vi "bone it.vi"() -> ()   [LabVIEW 2015]
panel:
  in  "milliseconds to wait 2":u32
  in  "milliseconds to wait":u32
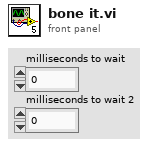
[diagram p1: front panel]
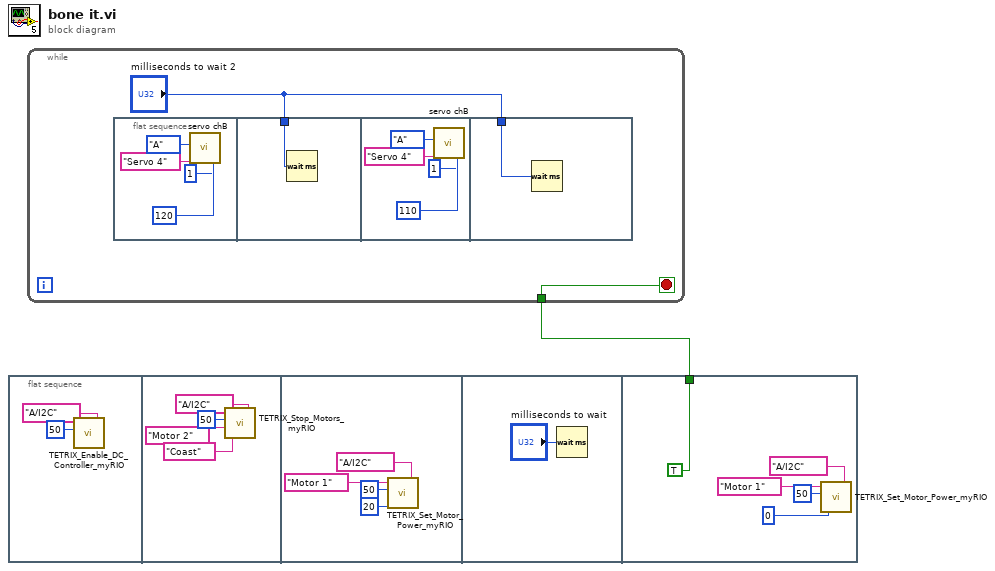
[diagram p0: block diagram]
diagram:
  n1 = flat-sequence {
    tunnel: [TRUE] -> w1
    frame #0 {
      n2 = call <vilib>:"TETRIX_Enable_DC_Controller_myRIO.vi"("myRIO MXP Port A/B"=tag "A/I2C", "Controller ID#  (I2C Address)"=u8 50) -> ()  [unwired: 5 in, 1 out]
    }
    frame #1 {
      n3 = call <vilib>:"TETRIX_Stop_Motors_myRIO.vi"("myRIO MXP Port A/B"=tag "A/I2C", "Stop Mode"="Coast", "Select Channel"="Motor 2", "Controller ID#  (I2C Address)"=u8 50) -> ()  [unwired: 3 in, 1 out]
    }
    frame #2 {
      n4 = call <vilib>:"TETRIX_Set_Motor_Power_myRIO.vi"("myRIO MXP Port A/B"=tag "A/I2C", "Power (-100 to 100)  0 = Coast Stop  125 = Brake Stop"=i8 20, "Select Channel"="Motor 1", "Controller ID#  (I2C Address)"=u8 50) -> ()  [unwired: 3 in, 1 out]
    }
    frame #3 {
      n5 = Wait (ms)(milliseconds to wait="milliseconds to wait") -> ()  [unwired: 1 out]
    }
    frame #4 {
      n6 = call <vilib>:"TETRIX_Set_Motor_Power_myRIO.vi"("myRIO MXP Port A/B"=tag "A/I2C", "Power (-100 to 100)  0 = Coast Stop  125 = Brake Stop"=i8 0, "Select Channel"="Motor 1", "Controller ID#  (I2C Address)"=u8 50) -> ()  [unwired: 3 in, 1 out]
    }
  }
  n7 = while {
    tunnel: w1 -> [w19]
    stop <- w19 stop-if-true
    n8 = flat-sequence {
      tunnel: "milliseconds to wait 2" -> [w24]
      tunnel: "milliseconds to wait 2" -> [w29]
      frame #0 {
        n9 = call "servo chB.vi"("Servo Position (0 - 255)"=u8 120, "Controller Daisy Chain Position (1 - 4)"=u8 1, "Select Servo"="Servo 4", "Enum"=enum16{"A", "B"}."A") -> ()  [unwired: 3 in, 1 out]
      }
      frame #1 {
        n10 = Wait (ms)(milliseconds to wait=w24) -> ()  [unwired: 1 out]
      }
      frame #2 {
        n11 = call "servo chB.vi"("Servo Position (0 - 255)"=u8 110, "Controller Daisy Chain Position (1 - 4)"=u8 1, "Select Servo"="Servo 4", "Enum"=enum16{"A", "B"}."A") -> ()  [unwired: 3 in, 1 out]
      }
      frame #3 {
        n12 = Wait (ms)(milliseconds to wait=w29) -> ()  [unwired: 1 out]
      }
    }
  }
